vi "HW_ni_Search Devcies in System.vi"() -> ()   [LabVIEW 2016]
uses:
  <resource>/objmgr/daqmx.rc
panel:
  out "DevNames":tag[](array[tag])
  out "数组 2":i32[](array[ring]) items=["M系列DAQ"=14643, "X系列DAQ"=15858, "E系列DAQ"=14642, "S系列DAQ"=14644, "B系列DAQ"=14662, "SC系列DAQ"=14645, "USB DAQ"=14646, "AO系列"=14647, "数字I/O"=14648, "TIO系列"=14661, "动态信号采集"=14649, "开关"=14650, "CompactDAQ机箱"=14658, "C系列模块"=14659, "SCXI模块"=14660, "SCC接线盒"=14704, "SCC模块"=14705, "NI ELVIS"=14755, "网络DAQ"=14829, "SC Express"=15886, "未知"=12588]
  in  "错误输入":errorcluster caption="错误输入（无错误）"
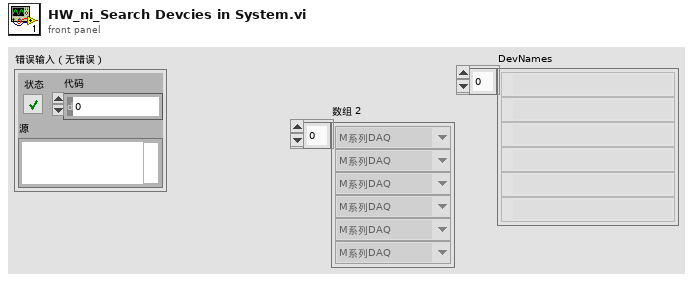
[diagram p1: front panel]
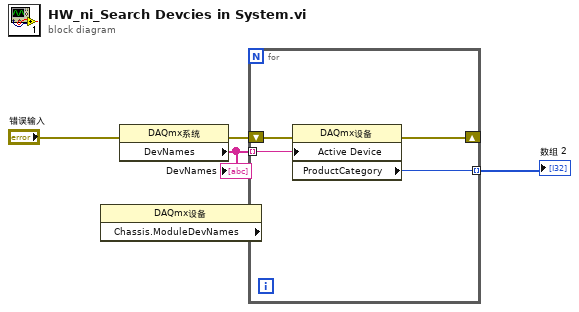
[diagram p0: block diagram]
diagram:
  n1 = property class="DAQmx设备" props=["Chassis.ModuleDevNames"]() -> ()  [unwired: 2 in, 3 out]
  n2 = property class="DAQmx系统"(error in="错误输入") -> (error out=w2:errorcluster, "DevNames"=w4:tag[])  [unwired: 1 in, 1 out]
  "DevNames" <- w4
  n3 = for {
    tunnel: w4 -> [w8] mode=indexing
    shift-right: [w6] -> _
    shift-left: w2 -> [w7]
    tunnel: [w5] -> w1 mode=indexing
    n4 = property class="DAQmx设备"(error in=w7, "Active Device"=w8) -> (error out=w6:errorcluster, "ProductCategory"=w5:i32)  [unwired: 1 in, 1 out]
  }
  "数组 2" <- w1
